vi "FPGA SPI_SPI Port.vi"(10 "Port":i8, 11 "FPGA IO":T1={"SCLK"="SCLK", "MOSI"="MOSI", "MISO"="MISO", "CS_0"="MISO", "CS_1"="MISO", "CS_2"="MISO", "CS_3"="MISO"}) -> ()   [LabVIEW 2015]
uses:
  Controls/FPGA SPI_Port_Info.ctl
  Controls/Port Action.ctl
  Controls/FPGA SPI_SPI Loop State.ctl
  <vilib>/Platform/TimedLoop/XDataNode/timing_clust.ctl
  <vilib>/Platform/TimedLoop/XDataNode/nitl_modes.ctl
  <vilib>/Platform/TimedLoop/XDataNode/wakeup.ctl
  <vilib>/rvi/Emulation/niFpgaGetClockAttributes.vi
  <vilib>/rvi/Emulation/niFpgaSctlEmulationGetInTimedLoop.vi
  <vilib>/rvi/Emulation/niFpgaEmulationReportErrorSimple.vi
  FPGA SPI_Globals.vi
  <vilib>/rvi/Emulation/niFpgaProcessEmulError.vi
  <vilib>/rvi/Emulation/niFpgaEmulationIsFPGAContextNoSignature.vi
  <vilib>/rvi/errors/niFpgaSetErrorForExecOnDevCompSimple.vi
  <vilib>/rvi/eio/common/nirviEmuReportErrorAndStop.vi
  <vilib>/rvi/DataTransferAndStorage/Container/Common/niFpgaContainerGetUniqueNameForEmu.vi
  <vilib>/rvi/FIFO/Fifo_Resource/nirvififoEmulationSetSize.vi
  <vilib>/rvi/FIFO/Fifo_Resource/nirviFifoEmulationQueueMgr.vi
  <instcachedir>/0/nirviFifoEmulationQueueMgr_E5CAEC123FF24DC58D834DCA3CDAA9B5.lvgen/nirviFifoEmulationQueueMgr_E5CAEC123FF24DC58D834DCA3CDAA9B5_002.vi
  <vilib>/Utility/error.llb/Clear Errors.vi
  <vilib>/rvi/FIFO/Fifo_Resource/nirvififoEmulationCreateLock.vi
  <vilib>/rvi/FIFO/Fifo_Resource/nirvififoEmulationObtainLock.vi
  <vilib>/rvi/FIFO/Fifo_Resource/nirvififoEmulationReleaseLock.vi
  <vilib>/rvi/occurrence/nirviWaitOnOccurrenceBase.vi
  <vilib>/rvi/errors/nirviReportUnexpectedCaseInternalError.vi
  <vilib>/rvi/errors/nirviReportUnexpectedCaseInternalError (U32).vi
  <vilib>/rvi/FIFO/Fifo_Resource/nirvififoEmulationDetermineInputValidOut.vi
  <vilib>/rvi/Emulation/niFpgaCriticalErrorInLSC.vi
  <vilib>/rvi/eio/common/nirviEmuTemplateMethod_errors.vi
  <vilib>/rvi/DataTransferAndStorage/Container/Common/niFpgaContainerSetEmuInfo.vi
  <vilib>/rvi/DataTransferAndStorage/Container/XNode/niFpgaContainer.xnode
  <vilib>/rvi/FIFO/Fifo_Resource/nirvififoEmulationRead.vi
  <vilib>/rvi/FIFO/Fifo_Resource/nirvififoEmulationWrite.vi
  <vilib>/Platform/TimedLoop/XDataNode/XDataNode.xnode
  <vilib>/eio/EIONode/EIONode.xnode
  <vilib>/rvi/LocalResourceManager/LocalResourceManager.xnode
  <vilib>/Platform/TimedLoop/XDataNode/XDNodeRunTimeDep.lvlib
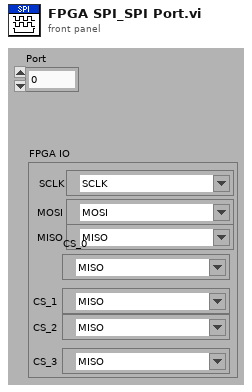
[diagram p1: front panel]
types:
  T1 = typedef "FPGA SPI_Port_Info.ctl" = cluster{"SCLK":refnum<k21>, "MOSI":refnum<k21>, "MISO":refnum<k21>, "CS_0":refnum<k21>, "CS_1":refnum<k21>, "CS_2":refnum<k21>, "CS_3":refnum<k21>}
  T2 = cluster{"CS":u8, "CS Active State":bool, "CPOL":bool, "CPHA":bool, "Wait Ticks":u32}
  T3 = typedef "Port Action.ctl" = enum8{"Idle", "Start", "Configure Hardware", "Start Hardware", "Set Done", "Wait Until Done"}
  T4 = typedef "FPGA SPI_SPI Loop State.ctl" = enum8{"Initialize", "Read From FIFO", "Set CS", "Wait Before Set", "Set Clock", "Wait Before Reset", "Reset Clock", "Write to FIFO", "Reset CS"}
  T5 = typedef "XDNodeRunTimeDep.lvlib/timing_clust.ctl" = cluster{"Expected End [f-1]":u64, "Actual End [f-1]":u64, "Finished Late? [f-1]":bool, "Expected End [i-1]":u64, "Actual End [i-1]":u64, "Finished Late? [i-1]":bool, "Expected Start [i]":u64, "Actual Start [i]":u64, "Expected Start [f]":u64, "Actual Start [f]":u64, "Source Name":string, "Structure Name":string, "Period":i64, "Deadline":i64, "Offset":i64, "Start":i64, "Priority":i32, "Timeout":i32, "Mode":T6, "Wakeup Reason":T7, "Error":errorcluster, "Source Type":string, "Secondary Source Type":string, "Global End Time":u64, "Global Start Time":u64, "Frame Duration":u64, "Iteration Duration":u64, "Assigned CPU":i32, "I/O Scan Engine Mode":u32}
  T6 = typedef "XDNodeRunTimeDep.lvlib/nitl_modes.ctl" = enum32{"No Change", "Process missed periods, maintain original phase", "Discard missed periods, maintain original phase", "Process missed periods, ignore original phase", "Discard missed periods, ignore original phase"}
  T7 = typedef "XDNodeRunTimeDep.lvlib/wakeup.ctl" = enum32{"Normal", "Aborted", "Asynchronous wakeup", "Timing source error", "Timed loop error", "Timeout"}
  T8 = typedef "FPGA SPI_FPGA SPI State.ctl" = enum8{"Idle", "Read/Write SPI", "Configure"}
  T9 = cluster{"MOSI":bool[], "MISO":bool[], "MOSI Byte Index":i8, "MISO Byte Index":i8}
  T10 = cluster{"Next State":T4, "Wait Count":u32, "Total Bits":u16, "Current Bit":u16, "Total Bytes":u16}
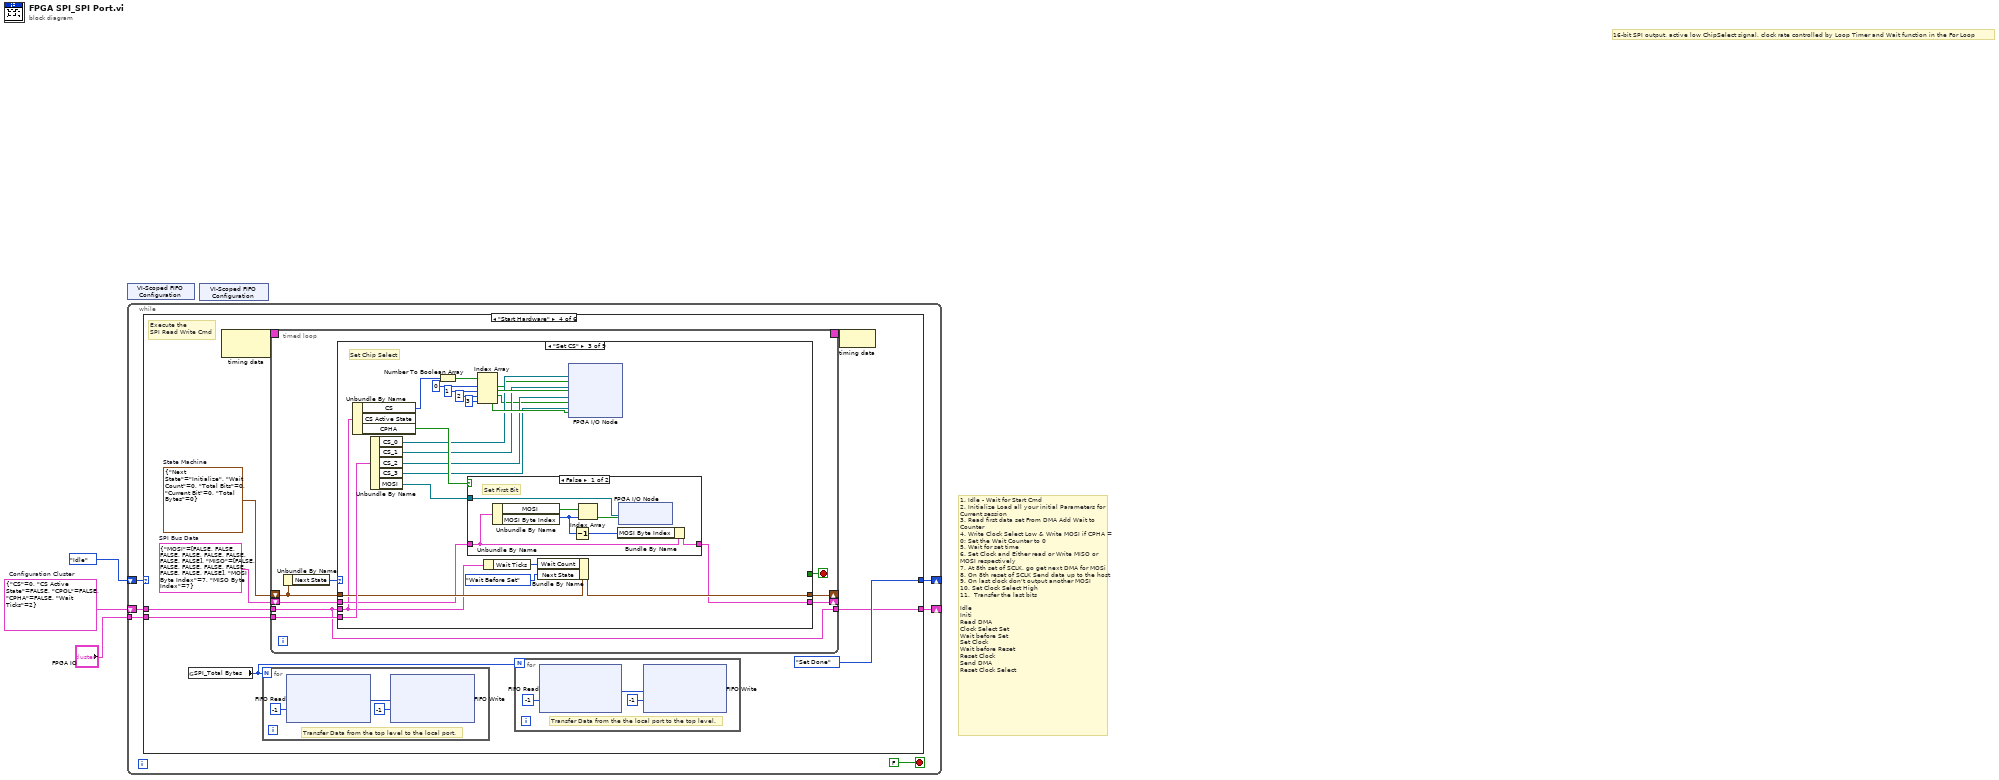
[diagram p0: block diagram]
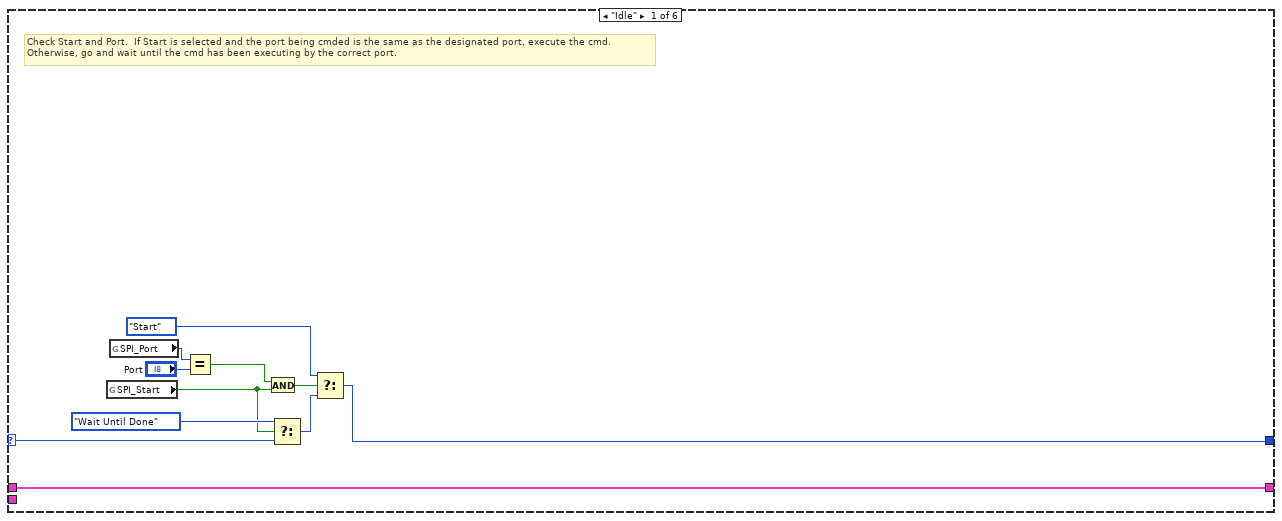
[diagram p2: hidden frame]
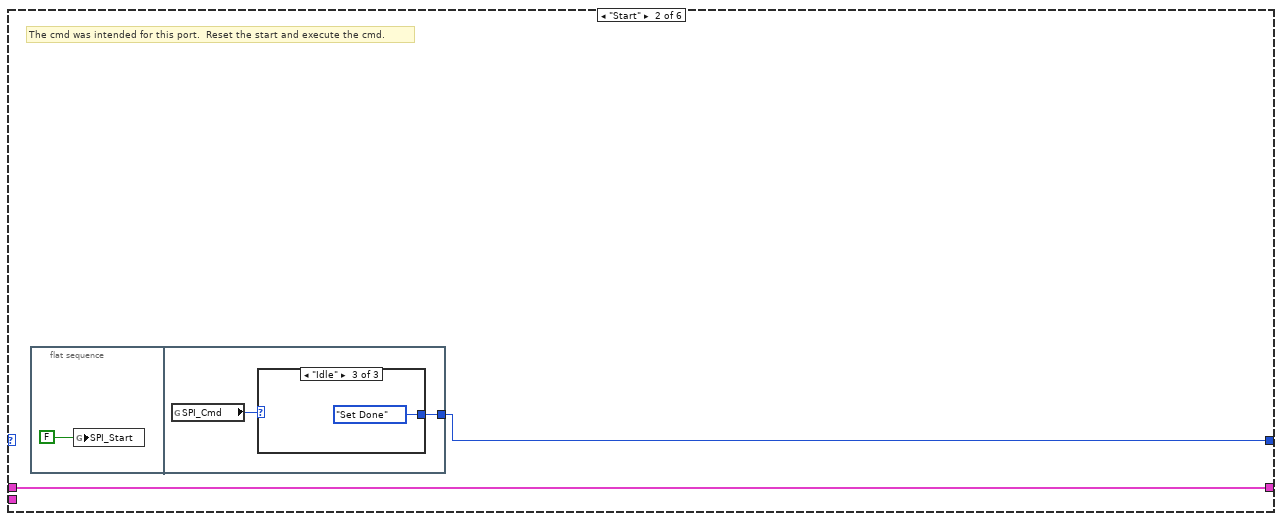
[diagram p3: hidden frame]
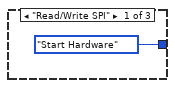
[diagram p4: hidden frame]
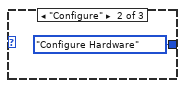
[diagram p5: hidden frame]
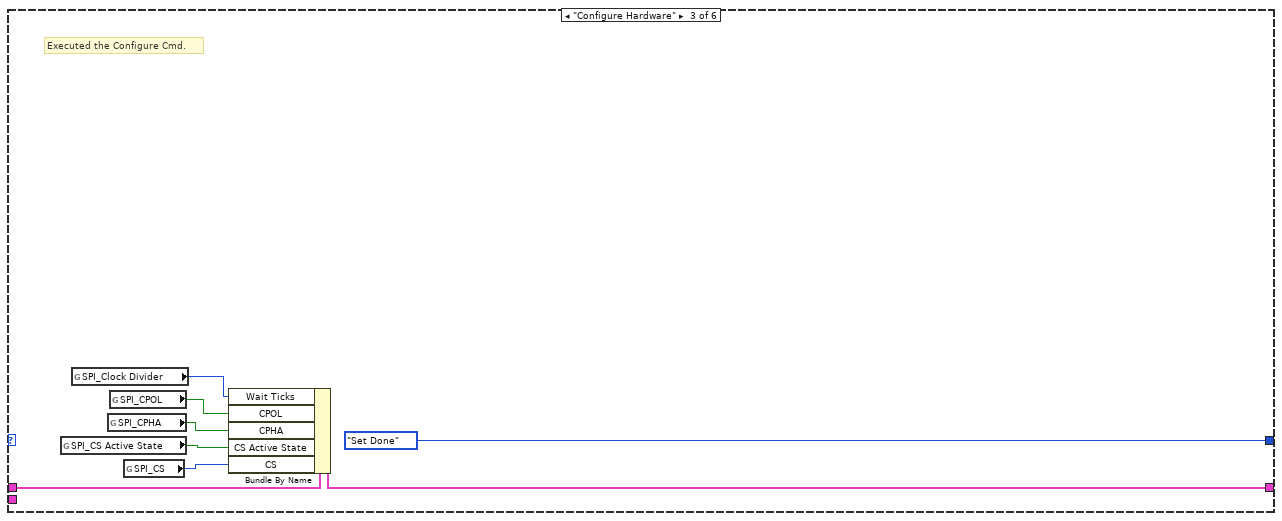
[diagram p6: hidden frame]
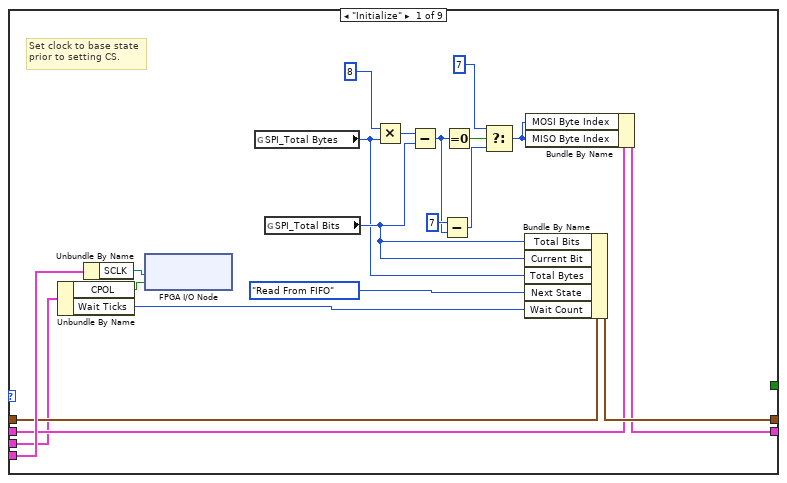
[diagram p7: hidden frame]
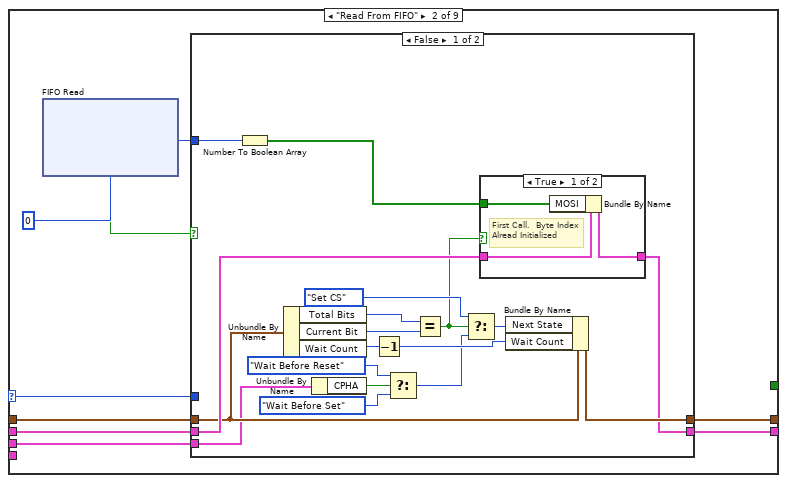
[diagram p8: hidden frame]
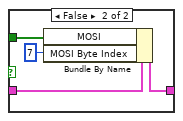
[diagram p9: hidden frame]
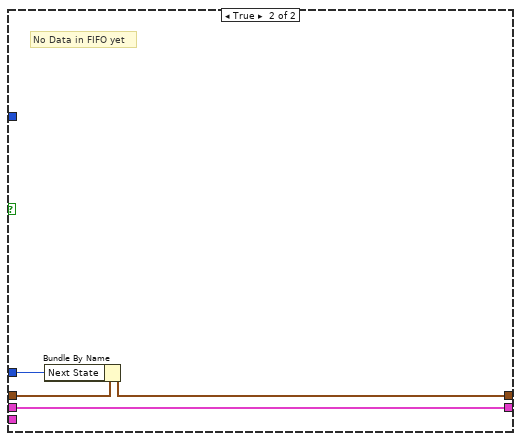
[diagram p10: hidden frame]
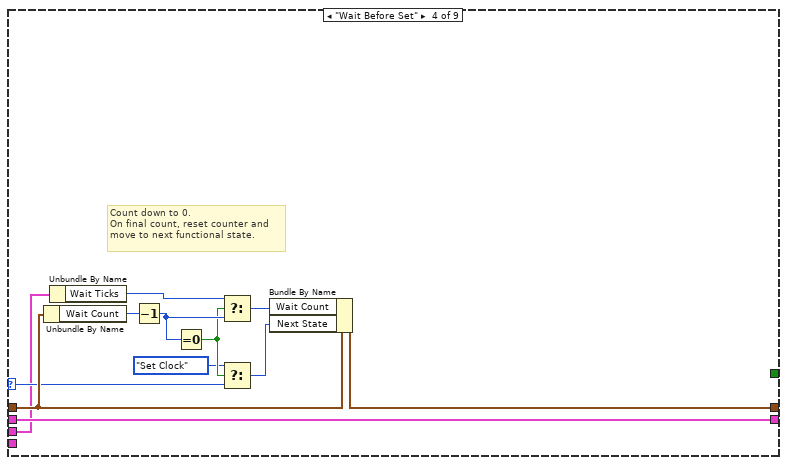
[diagram p12: hidden frame]
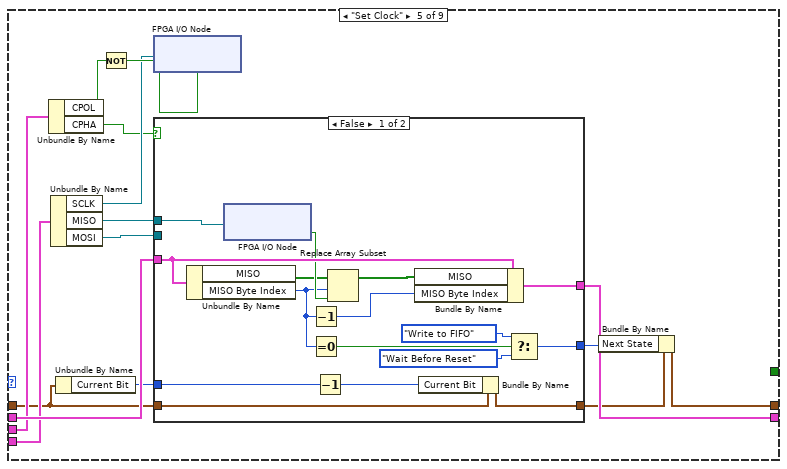
[diagram p13: hidden frame]
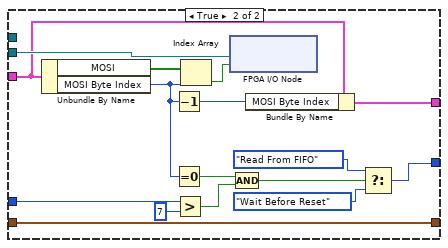
[diagram p14: hidden frame]
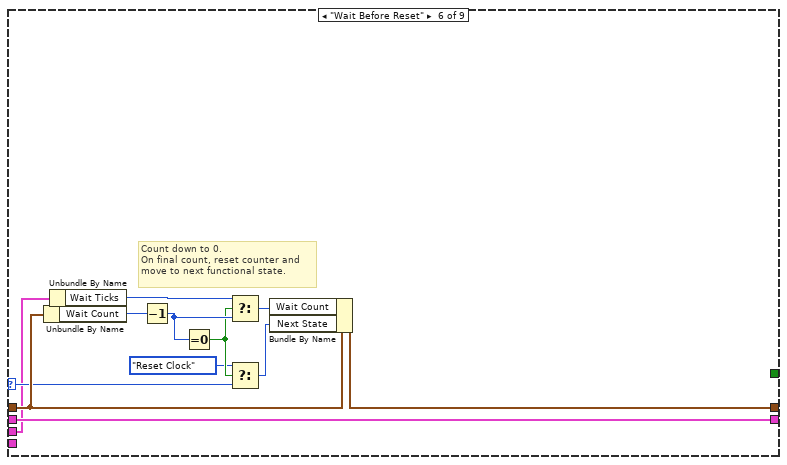
[diagram p15: hidden frame]
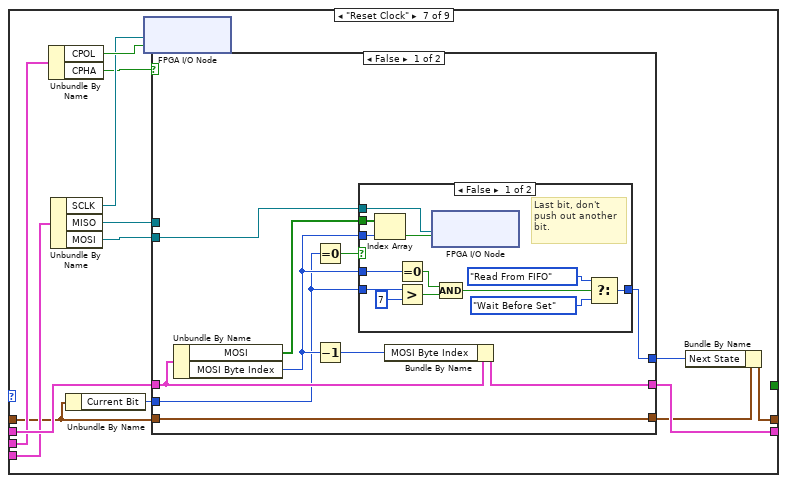
[diagram p16: hidden frame]
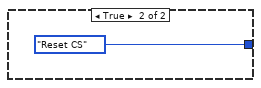
[diagram p17: hidden frame]
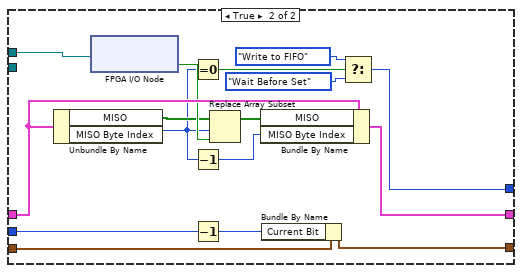
[diagram p18: hidden frame]
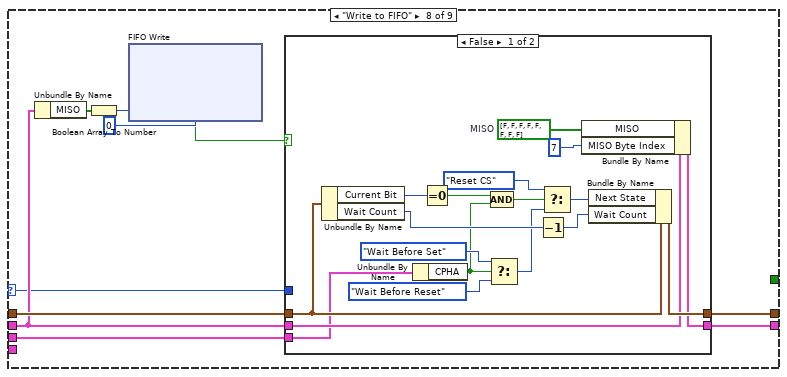
[diagram p19: hidden frame]
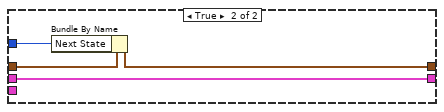
[diagram p20: hidden frame]
diagram:
  w2 = T2 {"CS"=0, "CS Active State"=FALSE, "CPOL"=FALSE, "CPHA"=FALSE, "Wait Ticks"=2}  # Configuration Cluster
  # "16-bit SPI output, active low ChipSelect signal, clock rate controlled by Loop Timer and Wait function in the For Loop"
  # "1. Idle - Wait for Start Cmd\n2. Initialize Load all your initial Parameters for Current session\n3. Read first data set From DMA Add Wait to Counter\n4. Write Clock Select Low & Write MOSI if CPHA = 0; Set the Wait Counter to 0\n5. Wait for set time\n6. Set Clock and Either read or Write MISO or MOSI respectively\n7. At 8th set of SCLK, go get next DMA for MOSi\n8. On 8th reset of SCLK Send data up to the host\n9. On last clock don't output another MOSI\n10. Set Clock Select High \n11.  Transfer the last bits\n\nIdle\nIniti\nRead DMA\nClock Select Set\nWait before Set\nSet Clock\nWait before Reset\nReset Clock\nSend DMA\nReset Clock Select"
  n1 = xnode "VI-Scoped FIFO Configuration"() -> ()  [unwired: 1 out]
  n2 = while {
    shift-right: [w8] -> _
    shift-left: Port_Action."Idle" ("Action") -> [w7]
    shift-right: [w4] -> _
    shift-left: w2 -> [w6]
    tunnel: "FPGA IO" -> [w5]
    stop <- FALSE stop-if-true
    n3 = case shown="\"Start Hardware\"" w7 {
      selector: w7 -> [w10 _ _ _ _ w329]
      tunnel: [w19 w22 Port_Action."Set Done" ("Action") Port_Action."Set Done" ("Action") Port_Action."Idle" ("Action") w328] -> w8
      tunnel: w6 -> [w14 w21 w32 w37 w324 w327]
      tunnel: w5 -> [_ _ _ w42 _ _]
      tunnel: [w14 w21 w31 w38 w324 w327] -> w4
      frame "Idle" {
        # "Check Start and Port.  If Start is selected and the port being cmded is the same as the designated port, execute the cmd.\nOtherwise, go and wait until the cmd has been executing by the correct port."
        n4 = global read "FPGA SPI_Globals.vi" "SPI_Start"() -> (w11:bool)
        n5 = global read "FPGA SPI_Globals.vi" "SPI_Port"() -> (w18:i8)
        n6 = Equal?(x=w18, y="Port") -> (x = y?=w12:bool)
        n7 = And(x=w12, y=w11) -> (x .and. y?=w16:bool)
        n8 = Select(t=Port_Action."Wait Until Done" ("Action"), s=w11, f=w10) -> (s? t:f=w15:T3)
        n9 = Select(t=Port_Action."Start" ("Action"), s=w16, f=w15) -> (s? t:f=w19:T3)
      }
      frame "Start" {
        # "The cmd was intended for this port.  Reset the start and execute the cmd."
        n10 = flat-sequence {
          tunnel: [w24] -> w22
          frame #0 {
            n11 = global write "FPGA SPI_Globals.vi" "SPI_Start"(FALSE ("Write Flag")) -> ()
          }
          frame #1 {
            n12 = global read "FPGA SPI_Globals.vi" "SPI_Cmd"() -> (w25:T8)
            n13 = case shown="\"Idle\"" w25 {
              tunnel: [Port_Action."Start Hardware" ("Action") Port_Action."Configure Hardware" ("Action") Port_Action."Set Done" ("Action")] -> w24
              frame "Read/Write SPI" {
              }
              frame "Configure" {
              }
              frame "Idle" {
              }
            }
          }
        }
      }
      frame "Configure Hardware" {
        # "Executed the Configure Cmd."
        n14 = global read "FPGA SPI_Globals.vi" "SPI_CS Active State"() -> (w34:bool)
        n15 = global read "FPGA SPI_Globals.vi" "SPI_Clock Divider"() -> (w29:u32)
        n16 = global read "FPGA SPI_Globals.vi" "SPI_CPHA"() -> (w33:bool)
        n17 = global read "FPGA SPI_Globals.vi" "SPI_CPOL"() -> (w36:bool)
        n18 = global read "FPGA SPI_Globals.vi" "SPI_CS"() -> (w35:u8)
        n19 = Bundle By Name(cluster=w32, "Wait Ticks"=w29, "CPOL"=w36, "CPHA"=w33, "CS Active State"=w34, "CS"=w35) -> (w31:T2)
      }
      frame "Start Hardware" {
        w40 = T9 {"MOSI"=[FALSE, FALSE, FALSE, FALSE, FALSE, FALSE, FALSE, FALSE], "MISO"=[FALSE, FALSE, FALSE, FALSE, FALSE, FALSE, FALSE, FALSE], "MOSI Byte Index"=7, "MISO Byte Index"=7}  # SPI Bus Data
        w41 = T10 {"Next State"=enum."Initialize", "Wait Count"=0, "Total Bits"=0, "Current Bit"=0, "Total Bytes"=0}  # State Machine
        # "Execute the \nSPI Read Write Cmd"
        n20 = global read "FPGA SPI_Globals.vi" "SPI_Total Bytes"() -> (w39:u16)
        n21 = node-c288() -> (w44:T5)  [unwired: 1 out]
        n22 = for {
          N: w39 -> [_]
          # "Transfer Data from the top level to the local port."
          n23 = xnode ("FIFO Read")("Timeout"=-1) -> ("Element"=w50:u8)  [unwired: 1 in, 2 out]
          n24 = xnode ("FIFO Write")("Element"=w50, "Timeout"=-1) -> ()  [unwired: 1 in, 2 out]
        }
        n25 = timed-loop {
          timing-out: [_] -> w43
          timing: w44 -> [_]
          shift-right: [w59] -> _
          shift-left: w41 -> [w58]
          shift-right: [w55] -> _
          shift-left: w40 -> [w56]
          tunnel: w42 -> [w53]
          tunnel: [w52] -> w38
          tunnel: w37 -> [w52]
          stop <- w54 stop-if-true
          n26 = Unbundle By Name(w58) -> ("Next State"=w57:T4)
          n27 = case shown="\"Set CS\"" w57 {
            selector: w57 -> [_ w80 _ w154 _ w212 _ w275 _]
            tunnel: w58 -> [w76 w83 w137 w160 w164 w219 w222 w281 w318]
            tunnel: [w75 w86 w141 w161 w176 w220 w234 w282 w319] -> w59
            tunnel: w52 -> [w61 w82 w132 w151 w171 w210 w230 w279 w315]
            tunnel: w56 -> [w62 w84 w134 w152 w172 w217 w232 w278 w316]
            tunnel: [w65 w85 w133 w152 w173 w217 w231 w277 w316] -> w55
            tunnel: w53 -> [w79 _ w140 _ w170 _ w229 _ w313]
            tunnel: [_ _ _ _ _ _ _ _ TRUE ("Start Hardware")] -> w54
            frame "Initialize" {
              # "Set clock to base state\nprior to setting CS."
              n28 = Unbundle By Name(w61) -> ("CPOL"=w77:bool, "Wait Ticks"=w60:u32)
              n29 = Unbundle By Name(w79) -> ("SCLK"=w78:refnum<k21>)
              n30 = xnode "FPGA I/O Node"("I/O Item"=w77, "FPGA I/O In"=w78) -> ()  [unwired: 1 out]
              n31 = global read "FPGA SPI_Globals.vi" "SPI_Total Bytes"() -> (w63:u16)
              n32 = global read "FPGA SPI_Globals.vi" "SPI_Total Bits"() -> (w64:u16)
              n33 = Multiply(x=u16 8 ("y"), y=w63) -> (x*y=w72:u16)
              n34 = Subtract(x=w72, y=w64) -> (x-y=w69:i8)
              n35 = Subtract(x=i8 7, y=w69) -> (x-y=w67:i8)
              n36 = Equal To 0?(x=w69) -> (x = 0?=w68:bool)
              n37 = Select(t=i8 7 ("y"), s=w68, f=w67) -> (s? t:f=w66:i8)
              n38 = Bundle By Name(cluster=w76, "Total Bits"=w64, "Current Bit"=w64, "Total Bytes"=w63, "Next State"=FPGA_SPI_SPI_Loop_State."Read From FIFO", "Wait Count"=w60) -> (w75:T10)
              n39 = Bundle By Name(cluster=w62, "MOSI Byte Index"=w66, "MISO Byte Index"=w66) -> (w65:T9)
            }
            frame "Read From FIFO" {
              n40 = xnode ("FIFO Read")("Timeout"=0) -> ("Element"=w87:u8, "Timed Out?"=w81:bool)  [unwired: 1 in, 1 out]
              n41 = case shown="False" w81 {
                tunnel: w87 -> [w106 _]
                tunnel: [w105 w114] -> w86
                tunnel: [w100 w117] -> w85
                tunnel: w84 -> [w99 w117]
                tunnel: w83 -> [w97 w115]
                tunnel: w82 -> [w89 _]
                tunnel: w80 -> [_ w116]
                frame False {
                  n42 = Number To Boolean Array(number=w106) -> (Boolean array=w98:bool[])
                  n43 = Unbundle By Name(w97) -> ("Total Bits"=w102:u16, "Current Bit"=w104:u16, "Wait Count"=w96:u32)
                  n44 = Unbundle By Name(w89) -> ("CPHA"=w93:bool)
                  n45 = Decrement(x=w96) -> (x-1=w95:u32)
                  n46 = Select(t=FPGA_SPI_SPI_Loop_State."Wait Before Reset" ("Next State"), s=w93, f=FPGA_SPI_SPI_Loop_State."Wait Before Set" ("Next State")) -> (s? t:f=w90:T4)
                  n47 = Equal?(x=w102, y=w104) -> (x = y?=w94:bool)
                  n48 = Select(t=FPGA_SPI_SPI_Loop_State."Set CS" ("Next State"), s=w94, f=w90) -> (s? t:f=w101:T4)
                  n49 = case shown="True" w94 {
                    tunnel: [w109 w113] -> w100
                    tunnel: w99 -> [w108 w112]
                    tunnel: w98 -> [w107 w111]
                    frame True {
                      # "First Call.  Byte Index Alread Initialized"
                      n50 = Bundle By Name(cluster=w108, "MOSI"=w107) -> (w109:T9)
                    }
                    frame False {
                      n51 = Bundle By Name(cluster=w112, "MOSI"=w111, "MOSI Byte Index"=i8 7) -> (w113:T9)
                    }
                  }
                  n52 = Bundle By Name(cluster=w97, "Next State"=w101, "Wait Count"=w95) -> (w105:T10)
                }
                frame True {
                  # "No Data in FIFO yet"
                  n53 = Bundle By Name(cluster=w115, "Next State"=w116) -> (w114:T10)
                }
              }
            }
            frame "Set CS" {
              # "Set Chip Select"
              n54 = Unbundle By Name(w132) -> ("CS"=w131:u8, "CPHA"=w138:bool)  [unwired: 1 out]
              n55 = Unbundle By Name(w140) -> ("CS_0"=w123:refnum<k21>, "CS_1"=w122:refnum<k21>, "CS_2"=w121:refnum<k21>, "CS_3"=w120:refnum<k21>, "MOSI"=w139:refnum<k21>)
              n56 = Number To Boolean Array(number=w131) -> (Boolean array=w130:bool[])
              n57 = case shown="False" w138 {
                tunnel: w134 -> [w144 w149]
                tunnel: w139 -> [w146 _]
                tunnel: [w142 w149] -> w133
                frame False {
                  # "Set First Bit"
                  n58 = Unbundle By Name(w144) -> ("MOSI"=w148:bool[], "MOSI Byte Index"=w145:i8)
                  n59 = Decrement(x=w145) -> (x-1=w143:i8)
                  n60 = Index Array(array=w148, index=w145) -> (element=w147:bool)
                  n61 = Bundle By Name(cluster=w144, "MOSI Byte Index"=w143) -> (w142:T9)
                  n62 = xnode "FPGA I/O Node"("I/O Item"=w147, "FPGA I/O In"=w146) -> ()  [unwired: 1 out]
                }
                frame True {
                }
              }
              n63 = Index Array(array=w130, index #1=0 ("index"), index #2=1 ("index"), index #3=2 ("index"), index #4=3 ("index")) -> (element #1=w119:bool, element #2=w125:bool, element #3=w118:bool, element #4=w124:bool)
              n64 = Unbundle By Name(w132) -> ("Wait Ticks"=w136:u32)
              n65 = Bundle By Name(cluster=w137, "Wait Count"=w136, "Next State"=FPGA_SPI_SPI_Loop_State."Wait Before Set" ("Enum")) -> (w141:T10)
              n66 = xnode "FPGA I/O Node"("I/O Item"=w119, "FPGA I/O In"=w123, "I/O Item"=w125, "FPGA I/O In"=w122, "I/O Item"=w118, "FPGA I/O In"=w121, "I/O Item"=w124, "FPGA I/O In"=w120) -> ()  [unwired: 4 out]
            }
            frame "Wait Before Set" {
              # "Count down to 0.\nOn final count, reset counter and\nmove to next functional state."
              n67 = Unbundle By Name(w160) -> ("Wait Count"=w158:u32)
              n68 = Unbundle By Name(w151) -> ("Wait Ticks"=w150:u32)
              n69 = Decrement(x=w158) -> (x-1=w159:u32)
              n70 = Equal To 0?(x=w159) -> (x = 0?=w157:bool)
              n71 = Select(t=w150, s=w157, f=w159) -> (s? t:f=w156:u32)
              n72 = Select(t=FPGA_SPI_SPI_Loop_State."Set Clock", s=w157, f=w154) -> (s? t:f=w155:T4)
              n73 = Bundle By Name(cluster=w160, "Wait Count"=w156, "Next State"=w155) -> (w161:T10)
            }
            frame "Set Clock" {
              n74 = Unbundle By Name(w171) -> ("CPOL"=w174:bool, "CPHA"=w166:bool)
              n75 = Unbundle By Name(w170) -> ("SCLK"=w167:refnum<k21>, "MISO"=w168:refnum<k21>, "MOSI"=w169:refnum<k21>)
              n76 = Unbundle By Name(w164) -> ("Current Bit"=w163:u16)
              n77 = Not(x=w174) -> (.not. x?=w175:bool)
              n78 = xnode "FPGA I/O Node"("I/O Item"=w175, "FPGA I/O In"=w167) -> ()  [unwired: 1 out]
              n79 = case shown="False" w166 {
                tunnel: [w192 w195] -> w173
                tunnel: w172 -> [w191 w196]
                tunnel: w169 -> [_ w206]
                tunnel: w168 -> [w186 _]
                tunnel: w164 -> [w185 w205]
                tunnel: [w184 w205] -> w165
                tunnel: w163 -> [w183 w203]
                tunnel: [w178 w197] -> w162
                frame False {
                  n80 = Unbundle By Name(w191) -> ("MISO"=w189:bool[], "MISO Byte Index"=w182:i8)
                  n81 = xnode "FPGA I/O Node"("FPGA I/O In"=w186) -> ("I/O Item"=w190:bool)  [unwired: 1 out]
                  n82 = Decrement(x=w182) -> (x-1=w187:i8)
                  n83 = Equal To 0?(x=w182) -> (x = 0?=w177:bool)
                  n84 = Decrement(x=w183) -> (x-1=w181:u16)
                  n85 = Replace Array Subset(array=w189, new element=w190, index=w182) -> (w188:bool[])
                  n86 = Bundle By Name(cluster=w191, "MISO"=w188, "MISO Byte Index"=w187) -> (w192:T9)
                  n87 = Bundle By Name(cluster=w185, "Current Bit"=w181) -> (w184:T10)
                  n88 = Select(t=FPGA_SPI_SPI_Loop_State."Write to FIFO" ("Enum"), s=w177, f=FPGA_SPI_SPI_Loop_State."Wait Before Reset" ("Enum")) -> (s? t:f=w178:T4)
                }
                frame True {
                  n89 = Unbundle By Name(w196) -> ("MOSI"=w208:bool[], "MOSI Byte Index"=w194:i8)
                  n90 = Decrement(x=w194) -> (x-1=w193:i8)
                  n91 = Equal To 0?(x=w194) -> (x = 0?=w204:bool)
                  n92 = Greater?(x=w203, y=u16 7 ("x")) -> (0:w201:bool)
                  n93 = Index Array(array=w208, index=w194) -> (element=w207:bool)
                  n94 = xnode "FPGA I/O Node"("I/O Item"=w207, "FPGA I/O In"=w206) -> ()  [unwired: 1 out]
                  n95 = Compound Arithmetic op=AND(w204, w201) -> (w200:bool)
                  n96 = Bundle By Name(cluster=w196, "MOSI Byte Index"=w193) -> (w195:T9)
                  n97 = Select(t=FPGA_SPI_SPI_Loop_State."Read From FIFO" ("Enum"), s=w200, f=FPGA_SPI_SPI_Loop_State."Wait Before Reset" ("Enum")) -> (s? t:f=w197:T4)
                }
              }
              n98 = Bundle By Name(cluster=w165, "Next State"=w162) -> (w176:T10)
            }
            frame "Wait Before Reset" {
              # "Count down to 0.\nOn final count, reset counter and\nmove to next functional state."
              n99 = Unbundle By Name(w219) -> ("Wait Count"=w216:u32)
              n100 = Unbundle By Name(w210) -> ("Wait Ticks"=w209:u32)
              n101 = Decrement(x=w216) -> (x-1=w218:u32)
              n102 = Equal To 0?(x=w218) -> (x = 0?=w215:bool)
              n103 = Select(t=w209, s=w215, f=w218) -> (s? t:f=w214:u32)
              n104 = Select(t=FPGA_SPI_SPI_Loop_State."Reset Clock", s=w215, f=w212) -> (s? t:f=w213:T4)
              n105 = Bundle By Name(cluster=w219, "Wait Count"=w214, "Next State"=w213) -> (w220:T10)
            }
            frame "Reset Clock" {
              n106 = Unbundle By Name(w230) -> ("CPOL"=w233:bool, "CPHA"=w225:bool)
              n107 = Unbundle By Name(w229) -> ("SCLK"=w226:refnum<k21>, "MISO"=w227:refnum<k21>, "MOSI"=w228:refnum<k21>)
              n108 = Unbundle By Name(w222) -> ("Current Bit"=w221:u16)
              n109 = xnode "FPGA I/O Node"("I/O Item"=w233, "FPGA I/O In"=w226) -> ()  [unwired: 1 out]
              n110 = case shown="False" w225 {
                tunnel: [w239 w270] -> w231
                tunnel: w232 -> [w240 w274]
                tunnel: w228 -> [w244 _]
                tunnel: w227 -> [_ w271]
                tunnel: w222 -> [w241 w268]
                tunnel: [w241 w267] -> w224
                tunnel: [w235 w261] -> w223
                tunnel: w221 -> [w236 w259]
                frame False {
                  n111 = Unbundle By Name(w240) -> ("MOSI"=w243:bool[], "MOSI Byte Index"=w237:i8)
                  n112 = Equal To 0?(x=w236) -> (x = 0?=w242:bool)
                  n113 = Decrement(x=w237) -> (x-1=w238:i8)
                  n114 = case shown="False" w242 {
                    tunnel: w244 -> [w256 _]
                    tunnel: w243 -> [w255 _]
                    tunnel: w237 -> [w254 _]
                    tunnel: w237 -> [w250 _]
                    tunnel: w236 -> [w249 _]
                    tunnel: [w245 FPGA_SPI_SPI_Loop_State."Reset CS" ("Enum")] -> w235
                    frame False {
                      # "Last bit, don't\npush out another\nbit."
                      n115 = Index Array(array=w255, index=w254) -> (element=w257:bool)
                      n116 = Equal To 0?(x=w250) -> (x = 0?=w252:bool)
                      n117 = Greater?(x=w249, y=u16 7 ("x")) -> (0:w253:bool)
                      n118 = xnode "FPGA I/O Node"("I/O Item"=w257, "FPGA I/O In"=w256) -> ()  [unwired: 1 out]
                      n119 = Compound Arithmetic op=AND(w252, w253) -> (w246:bool)
                      n120 = Select(t=FPGA_SPI_SPI_Loop_State."Read From FIFO" ("Enum"), s=w246, f=FPGA_SPI_SPI_Loop_State."Wait Before Set" ("Enum")) -> (s? t:f=w245:T4)
                    }
                    frame True {
                    }
                  }
                  n121 = Bundle By Name(cluster=w240, "MOSI Byte Index"=w238) -> (w239:T9)
                }
                frame True {
                  n122 = Unbundle By Name(w274) -> ("MISO"=w272:bool[], "MISO Byte Index"=w263:i8)
                  n123 = xnode "FPGA I/O Node"("FPGA I/O In"=w271) -> ("I/O Item"=w273:bool)  [unwired: 1 out]
                  n124 = Equal To 0?(x=w263) -> (x = 0?=w260:bool)
                  n125 = Decrement(x=w263) -> (x-1=w266:i8)
                  n126 = Decrement(x=w259) -> (x-1=w262:u16)
                  n127 = Replace Array Subset(array=w272, new element=w273, index=w263) -> (w269:bool[])
                  n128 = Bundle By Name(cluster=w274, "MISO"=w269, "MISO Byte Index"=w266) -> (w270:T9)
                  n129 = Bundle By Name(cluster=w268, "Current Bit"=w262) -> (w267:T10)
                  n130 = Select(t=FPGA_SPI_SPI_Loop_State."Write to FIFO" ("Enum"), s=w260, f=FPGA_SPI_SPI_Loop_State."Wait Before Set" ("Enum")) -> (s? t:f=w261:T4)
                }
              }
              n131 = Bundle By Name(cluster=w224, "Next State"=w223) -> (w234:T10)
            }
            frame "Write to FIFO" {
              n132 = Unbundle By Name(w278) -> ("MISO"=w284:bool[])
              n133 = Boolean Array To Number(Boolean array=w284) -> (number=w283:u8)
              n134 = xnode ("FIFO Write")("Element"=w283, "Timeout"=0) -> ("Timed Out?"=w276:bool)  [unwired: 1 in, 1 out]
              n135 = case shown="False" w276 {
                tunnel: [w302 w304] -> w282
                tunnel: w281 -> [w301 w305]
                tunnel: w279 -> [w285 _]
                tunnel: w278 -> [w288 w306]
                tunnel: [w286 w306] -> w277
                tunnel: w275 -> [_ w303]
                frame False {
                  w289 = bool[] [FALSE, FALSE, FALSE, FALSE, FALSE, FALSE, FALSE, FALSE]  # MISO
                  n136 = Unbundle By Name(w301) -> ("Current Bit"=w300:u16, "Wait Count"=w297:u32)
                  n137 = Unbundle By Name(w285) -> ("CPHA"=w291:bool)
                  n138 = Equal To 0?(x=w300) -> (x = 0?=w293:bool)
                  n139 = Select(t=FPGA_SPI_SPI_Loop_State."Wait Before Set" ("Next State"), s=w291, f=FPGA_SPI_SPI_Loop_State."Wait Before Reset" ("Next State")) -> (s? t:f=w294:T4)
                  n140 = Compound Arithmetic op=AND(w293, w291) -> (w292:bool)
                  n141 = Decrement(x=w297) -> (x-1=w290:u32)
                  n142 = Select(t=FPGA_SPI_SPI_Loop_State."Reset CS" ("Next State"), s=w292, f=w294) -> (s? t:f=w298:T4)
                  n143 = Bundle By Name(cluster=w288, "MISO"=w289, "MISO Byte Index"=i8 7) -> (w286:T9)
                  n144 = Bundle By Name(cluster=w301, "Next State"=w298, "Wait Count"=w290) -> (w302:T10)
                }
                frame True {
                  n145 = Bundle By Name(cluster=w305, "Next State"=w303) -> (w304:T10)
                }
              }
            }
            frame "Reset CS" {
              # "Reset all CS signals.  Stop the loop."
              n146 = Unbundle By Name(w315) -> ("CS Active State"=w314:bool)
              n147 = Unbundle By Name(w313) -> ("CS_0"=w311:refnum<k21>, "CS_1"=w310:refnum<k21>, "CS_2"=w309:refnum<k21>, "CS_3"=w308:refnum<k21>)
              n148 = Not(x=w314) -> (.not. x?=w307:bool)
              n149 = Bundle By Name(cluster=w318, "Next State"=FPGA_SPI_SPI_Loop_State."Initialize" ("Enum")) -> (w319:T10)
              n150 = xnode "FPGA I/O Node"("I/O Item"=w307, "FPGA I/O In"=w311, "I/O Item"=w307, "FPGA I/O In"=w310, "I/O Item"=w307, "FPGA I/O In"=w309, "I/O Item"=w307, "FPGA I/O In"=w308) -> ()  [unwired: 4 out]
            }
          }
        }
        n151 = for {
          N: w39 -> [_]
          # "Transfer Data from the the local port to the top level."
          n152 = xnode ("FIFO Read")("Timeout"=-1) -> ("Element"=w47:u8)  [unwired: 1 in, 2 out]
          n153 = xnode ("FIFO Write")("Element"=w47, "Timeout"=-1) -> ()  [unwired: 1 in, 2 out]
        }
        n154 = node-c288(w43) -> ()
      }
      frame "Set Done" {
        # "Set the done flag"
        n155 = global write "FPGA SPI_Globals.vi" "SPI_Done"(TRUE ("Done")) -> ()
      }
      frame "Wait Until Done" {
        # "Wait until the executing port finishes."
        n156 = global read "FPGA SPI_Globals.vi" "SPI_Done"() -> (w331:bool)
        n157 = Select(t=Port_Action."Idle" ("Action"), s=w331, f=w329) -> (s? t:f=w328:T3)
      }
    }
  }
  n158 = xnode "VI-Scoped FIFO Configuration"() -> ()  [unwired: 1 out]
